vi "Read P (mb).vi"(8 "error in (no error)":errorcluster, 11 "Gas Properties in":refnum<class "Gas Properties.lvclass">) -> (0 "error out":errorcluster, 2 "P (mb)":dbl, 3 "Gas Properties out":refnum<class "Gas Properties.lvclass">)   [LabVIEW 2015, in "Gas Properties.lvclass"]
uses:
  Gas Properties.lvclass
  Gas Properties.lvclass/Gas Properties.ctl
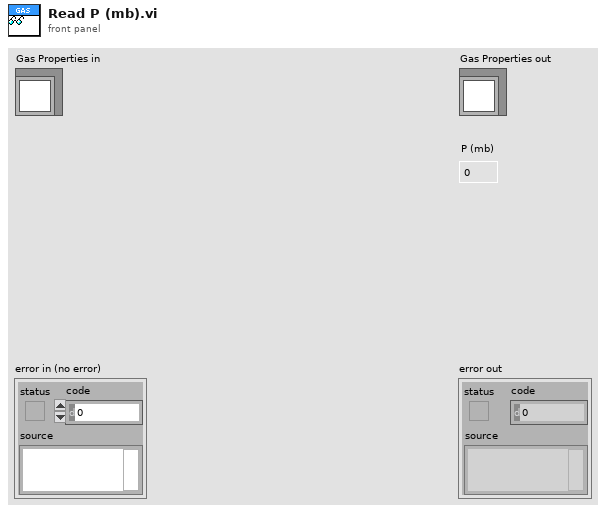
[diagram p1: front panel]
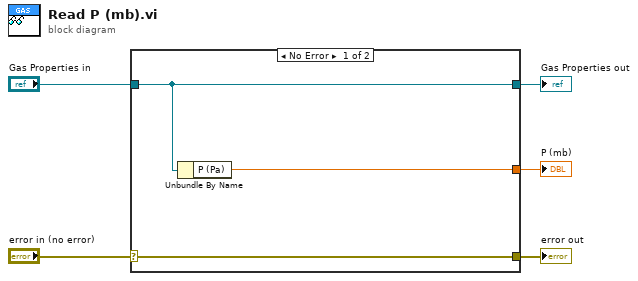
[diagram p0: block diagram]
diagram:
  n1 = case shown="No Error" "error in (no error)" {
    selector: "error in (no error)" -> [w8 w9]
    tunnel: [w8 w9] -> w4
    tunnel: [w7 w10] -> w2
    tunnel: "Gas Properties in" -> [w7 w10]
    tunnel: [w6 _] -> w1
    frame No Error {
      n2 = Unbundle By Name(w7) -> ("P (Pa)"=w6:dbl)
    }
    frame Error {
    }
  }
  "error out" <- w4
  "Gas Properties out" <- w2
  "P (mb)" <- w1
